vi "FTW-JSON-CompareEquality.vi"(0 "JSON":string, 5 "JSON to Compare":string, 11 "error in":errorcluster) -> (6 "Equal?":bool, 15 "error out":errorcluster)   [LabVIEW 2015]
uses:
  container/FTW-Container.lvclass
panel:
  # "Inputs"
  # "Outputs"
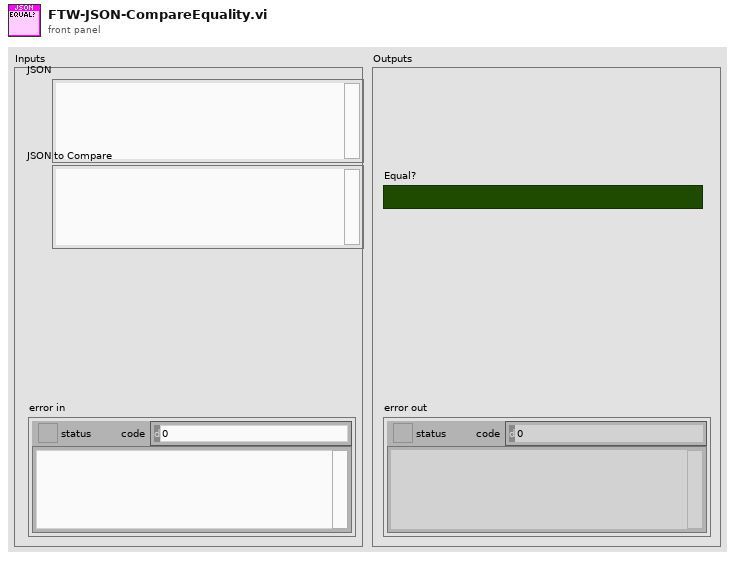
[diagram p1: front panel]
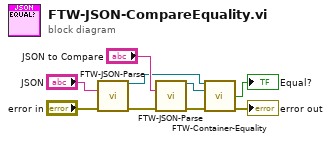
[diagram p0: block diagram]
diagram:
  n1 = call "FTW-JSON-Parse.vi"("JSON String"="JSON", "error in"="error in") -> ("Container"=w3:refnum<class "FTW-Container.lvclass">, "error out"=w8:errorcluster)  [unwired: 12 in]
  n2 = call "FTW-JSON-Parse.vi"("JSON String"="JSON to Compare", "error in"=w8) -> ("Container"=w2:refnum<class "FTW-Container.lvclass">, "error out"=w5:errorcluster)  [unwired: 12 in]
  n3 = call "FTW-Container-Equality.vi"("FTW-Container In"=w3, "Other Container"=w2, "error in"=w5) -> ("Equal"=→"Equal?":bool, "error out"=→"error out":errorcluster)  [unwired: 10 in, 1 out]
